vi "ImageGetData.vi"(8 "error in (no error)":errorcluster, 9 "Stage Position (mm)":dbl, 10 "Intensity Data":dbl[][](array[numeric]), 11 "Image in":refnum<class "Image.lvclass">) -> (0 "error out":errorcluster, 3 "Image out":refnum<class "Image.lvclass">)   [LabVIEW 2012, in "Image.lvclass"]
uses:
  classes/Image.lvclass
  classes/Image.lvclass/Image.ctl
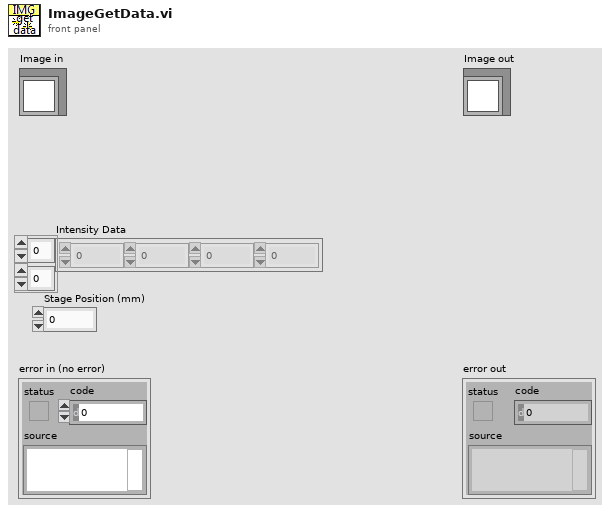
[diagram p1: front panel]
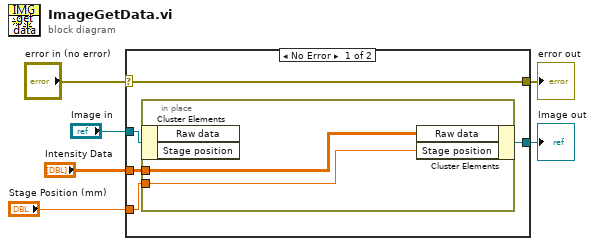
[diagram p0: block diagram]
diagram:
  n1 = case shown="No Error" "error in (no error)" {
    selector: "error in (no error)" -> [w11 w15]
    tunnel: [w11 w15] -> w5
    tunnel: [w7 w14] -> w3
    tunnel: "Image in" -> [w10 w14]
    tunnel: "Intensity Data" -> [w9 _]
    tunnel: "Stage Position (mm)" -> [w8 _]
    frame No Error {
      n2 = in-place {
        in-place-border: w9 -> [w13]
        in-place-border: w8 -> [w12]
        n3 = in-place-cluster #1(w10) -> ()  [unwired: 2 out]
        n4 = in-place-cluster #1("Raw data"=w13, "Stage position"=w12) -> (w7:refnum<class "Image.lvclass">)
      }
    }
    frame Error {
    }
  }
  "error out" <- w5
  "Image out" <- w3
